vi "Blinking test.vi"() -> ()   [LabVIEW 2016]
uses:
  Typedefs/ROB display info.ctl
  <vilib>/Utility/miscctls.llb/LVRowAndColumnTypeDef.ctl
panel:
  out "error out":errorcluster
  in  "stop":bool
  out "ROB Info-display":T1={"ID:"=-1, "State:"="UNKNOWN", "Voltages"=0, "Temp:"=-1.0, "Latch count:"=-1, "VRef:"=enum."Unknown", "Trigthres:"=-1, "MPPC EN"=FALSE, "Test charge"=FALSE, "Responding"=FALSE, "Last update"=timestamp(0 s since 1904-01-01)} {"Last update" format="%<%X>T"; "Trigthres:" format="%.0fmV"; "Temp:" format="%.2f C"}
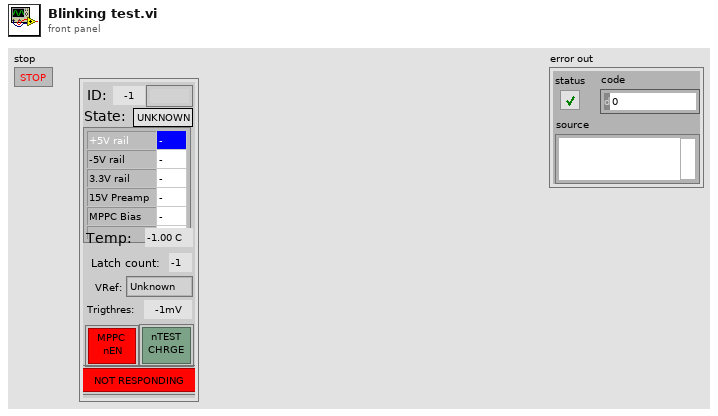
[diagram p1: front panel]
types:
  T1 = typedef "ROB display info.ctl" = cluster{"ID:":i32, "State:":string, "Voltages":i32, "Temp:":dbl, "Latch count:":i32, "VRef:":enum16{"External", "Internal", "Unknown"}, "Trigthres:":i32, "MPPC EN":bool, "Test charge":bool, "Responding":bool, "Last update":timestamp}
  T2 = typedef "LVRowAndColumnTypeDef.ctl" = cluster{"Row":i32, "Column":i32}
  T3 = enum16{"ID", "Status", "Voltages", "Temp", "Latch count", "VRef", "Trigthres", "MPPC EN?", "Test charge?", "Responding?"}
  T4 = typedef "ROB info refnum.ctl" = refnum<vi>
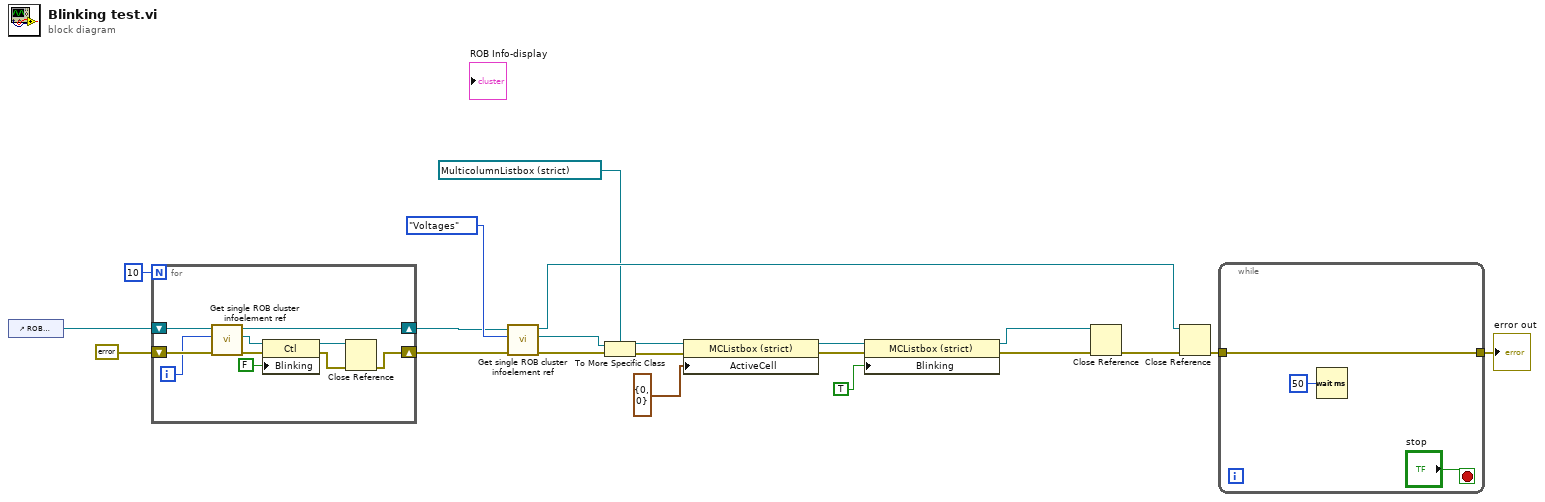
[diagram p0: block diagram]
diagram:
  n1 = control-ref of="ROB Info-display"() -> (w10:refnum<vi>)
  n2 = for {
    N: 10 -> [_]
    shift-right: [w22] -> w7
    shift-left: errorcluster {"status"=FALSE, "code"=0, "source"=""} ("error out") -> [w30]
    shift-right: [w25] -> w8
    shift-left: w10 -> [w31]
    i -> [w29]
    n3 = call "Get single ROB cluster infoelement ref.vi"("error in (no error)"=w30, "Enum"=w29, "ROB infocluster ref"=w31) -> ("error out"=w28:errorcluster, "Element reference"=w27:refnum<vi>, "ROB infocluster ref"=w25:T4)  [unwired: 6 in]
    n4 = property class="Ctl"(reference=w27, error in=w28, "Blinking"=FALSE) -> (reference out=w23:refnum<vi>, error out=w24:errorcluster)
    n5 = Close Reference(reference=w23, error in (no error)=w24) -> (error out=w22:errorcluster)
  }
  n6 = call "Get single ROB cluster infoelement ref.vi"("error in (no error)"=w7, "Enum"=T3."Voltages", "ROB infocluster ref"=w8) -> ("error out"=w15:errorcluster, "Element reference"=w16:refnum<vi>, "ROB infocluster ref"=w20:T4)  [unwired: 6 in]
  n7 = To More Specific Class(target class=refnum<vi> refnum ("Voltages"), reference=w16, error in=w15) -> (specific class reference=w13:refnum<vi>, error out=w14:errorcluster)
  n8 = property class="MCListbox (strict)"(reference=w13, error in=w14, "ActiveCell"=T2 {"Row"=0, "Column"=0} ("Active Cell:Active Cell")) -> (reference out=w3:refnum<vi>, error out=w5:errorcluster)
  n9 = property class="MCListbox (strict)"(reference=w3, error in=w5, "Blinking"=TRUE) -> (reference out=w1:refnum<vi>, error out=w4:errorcluster)
  n10 = Close Reference(reference=w1, error in (no error)=w4) -> (error out=w21:errorcluster)
  n11 = Close Reference(reference=w20, error in (no error)=w21) -> (error out=w19:errorcluster)
  n12 = while {
    tunnel: w19 -> [w34]
    tunnel: [w34] -> w18
    stop <- "stop" stop-if-true
    n13 = Wait (ms)(milliseconds to wait=u32 50) -> ()  [unwired: 1 out]
  }
  "error out" <- w18
